vi "ellie_test.vi"() -> ()   [LabVIEW 2009]
uses:
  <vilib>/Analysis/NI_AALBase.lvlib
panel:
  out "Q Meter - Raw":cluster{"Y":dbl[], "Y":dbl[]}[](graph)
  in  "On Switch":bool=TRUE
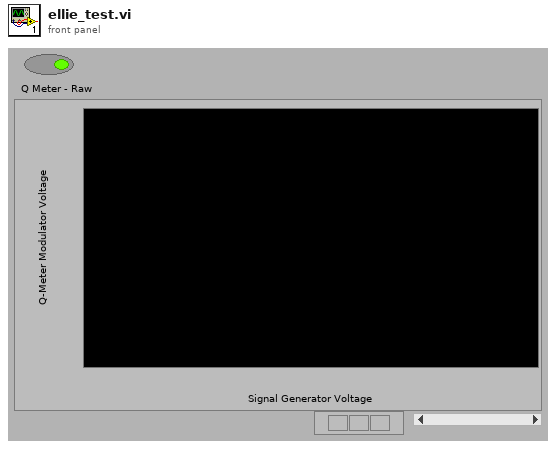
[diagram p1: front panel]
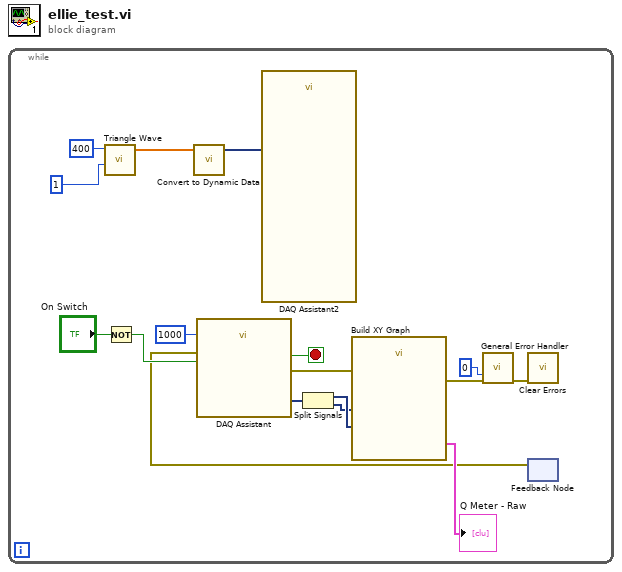
[diagram p0: block diagram]
diagram:
  n1 = while {
    stop <- w18 stop-if-true
    n2 = call <vilib>:"Triangle Wave.vi"("samples"=400, "frequency"=1) -> ("triangle wave"=w3:dbl[])  [unwired: 3 in, 2 out]
    n3 = Not(x="On Switch") -> (.not. x?=w7:bool)
    n4 = call "Convert to Dynamic Data"("Array"=w3) -> ("Dynamic Data Type"=w4:dynamicdata)  [unwired: 3 in]
    n5 = call "DAQ Assistant2"("data"=w4) -> ()  [unwired: 16 in, 3 out]
    n6 = feedback #1() -> (w5:errorcluster)  [unwired: 1 in]
    n7 = call "DAQ Assistant"("number of samples"=1000, "error in"=w5, "stop (F)"=w7) -> ("data"=w14:dynamicdata, "stopped"=w18:bool, "error out"=w12:errorcluster)  [unwired: 13 in, 1 out]
    n8 = Split Signals(w14) -> (w16:dynamicdata, w15:dynamicdata)  [unwired: 2 in]
    n9 = call "Build XY Graph"("error in (no error)"=w12, "Y Input"=w16, "X Input"=w15) -> ("error out"=w9:errorcluster, "XY Graph"=→"Q Meter - Raw":cluster{"Y":dbl[], "Y":dbl[]}[])  [unwired: 7 in]
    n10 = call <vilib>:"General Error Handler.vi"("type of dialog (OK msg:1)"=0, "error in (no error)"=w9) -> ("error out"=w10:errorcluster)  [unwired: 9 in, 4 out]
    n11 = call <vilib>:"Clear Errors.vi"("error in (no error)"=w10) -> ("error out"=w6:errorcluster)  [unwired: 6 in]
  }
